vi "(SubVI) Pull DNA_ver2_YCC.vi"(0 "waiting time per point (ms)\nrange from 5ms to 0.167 ms":dbl=0.5, 1 "Filter type":T1(ring), 2 "Avg points":i32, 3 "Real initial position (um)":dbl format="%0.5f", 5 "Record?":bool, 7 "T=X\nF=Y":bool, 9 "Toward  ?\nT=+, F=-":bool, 11 "no Record scan rate  (um/s)":dbl=2.0, 12 "Record scan rate  (um/s)":dbl=2.0 format="%.3f", 13 "range  (um)":dbl=2.0 min=0.0 max=100.0 step=0.5 format="%.3f", 14 "Sampling rate":dbl=20000.0 format="%0.2f") -> (4 "True rate?":bool, 6 "Raw Stage Array":dbl[](array[numeric]), 8 "Filtered Stage Array":dbl[](array[numeric]) format="%0.2f", 10 "Filtered QPD Array":dbl[](array[numeric]) format="%0.2f")   [LabVIEW 2014]
panel:
  out "delay (ms)":dbl
  out "scan rate  (um/s)":dbl
  out "axis":u32=1
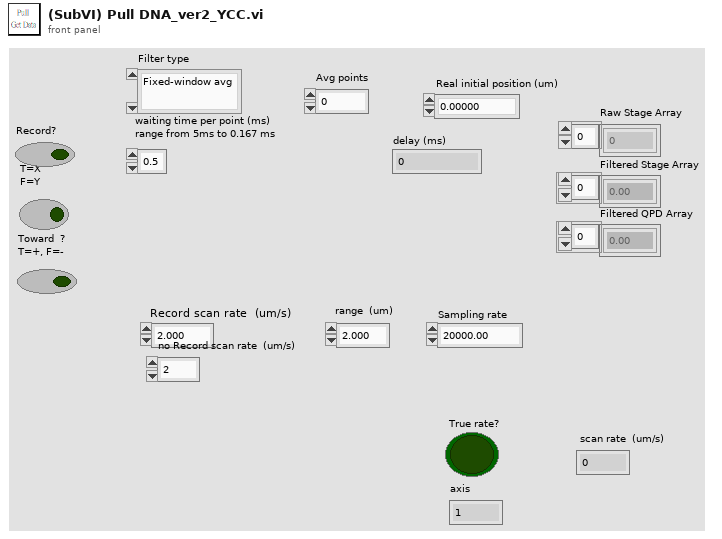
[diagram p1: front panel]
types:
  T1 = enum16{"Fixed-window avg", "Moving-window avg", "F+S-window avg", "S-G filter", "Fixed-window Median", "Moving-window Median "}
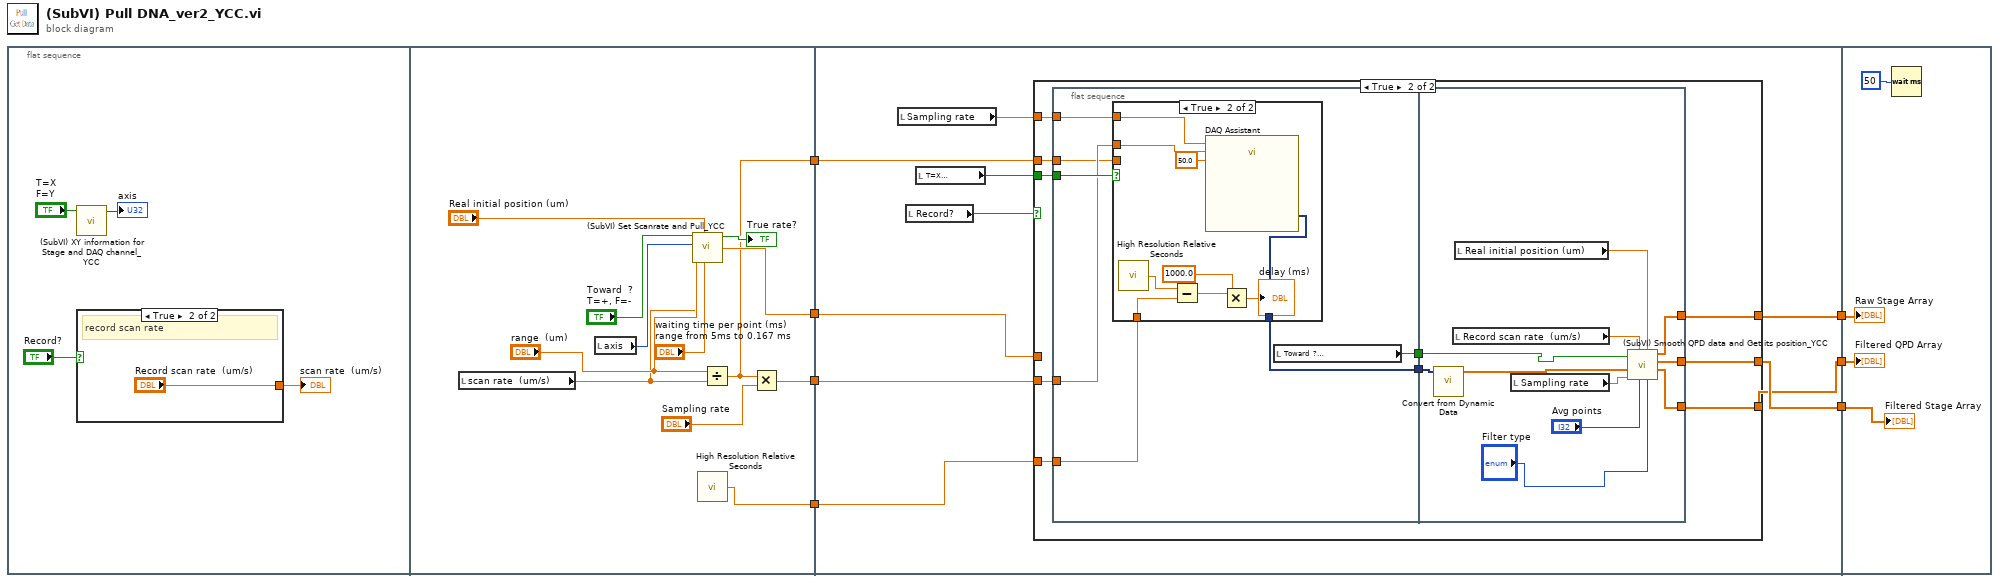
[diagram p0: block diagram]
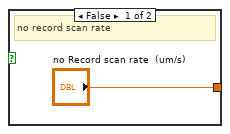
[diagram p2: hidden frame]
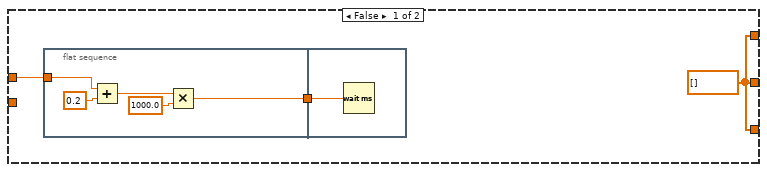
[diagram p3: hidden frame]
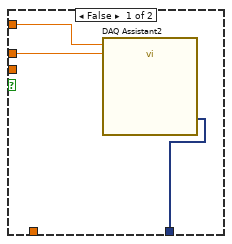
[diagram p4: hidden frame]
diagram:
  n1 = flat-sequence {
    tunnel: [w23] -> w4
    tunnel: [w17] -> w3
    tunnel: [w16] -> w2
    tunnel: [w14] -> w1
    tunnel: [w33] -> w7
    tunnel: [w32] -> w6
    tunnel: [w31] -> w5
    tunnel: w2 -> [w27]
    tunnel: w3 -> [w28]
    tunnel: w4 -> [w35]
    tunnel: w1 -> [w26]
    tunnel: w7 -> [w88]
    tunnel: w6 -> [w87]
    tunnel: w5 -> [w86]
    frame #0 {
      n2 = call "(SubVI) XY information for Stage and DAQ channel_YCC.vi"("T=X\nF=Y"="T=X\nF=Y") -> ("Axis"=→"axis":i32)  [unwired: 3 in, 1 out]
      n3 = case shown="True" "Record?" {
        tunnel: ["no Record scan rate  (um/s)" "Record scan rate  (um/s)"] -> w8
        frame False {
          # "no record scan rate"
        }
        frame True {
          # "record scan rate"
        }
      }
      "scan rate  (um/s)" <- w8
    }
    frame #1 {
      n4 = local read "scan rate  (um/s)"() -> (w18:dbl)
      n5 = local read "axis"() -> (w24:u32)
      n6 = call "(SubVI) Set Scanrate and Pull_YCC.vi"("toward+ ?\nT=+, F=-"="Toward  ?\nT=+, F=-", "Start From  (um)"="Real initial position (um)", "axis"=w24, "scan rate  (um/s)"=w18, "waiting time per point (ms)\nrange from 5ms to 0.167 ms"="waiting time per point (ms)\nrange from 5ms to 0.167 ms", "range  (um)"="range  (um)") -> ("True rate?"=→"True rate?":bool, "traveling time (s)"=w17:dbl)  [unwired: 1 out]
      n7 = call <vilib>:"High Resolution Relative Seconds.vi"() -> ("relative seconds"=w14:dbl)
      n8 = Divide(x="range  (um)", y=w18) -> (x/y=w16:dbl)
      n9 = Multiply(x=w16, y="Sampling rate") -> (x*y=w23:dbl)
    }
    frame #2 {
      n10 = local read "Sampling rate"() -> (w29:dbl)
      n11 = local read "Record?"() -> (w34:bool)
      n12 = local read "T=X\nF=Y"() -> (w30:bool)
      n13 = case shown="True" w34 {
        tunnel: w35 -> [_ w54]
        tunnel: [w38 w51] -> w33
        tunnel: [w38 w50] -> w31
        tunnel: [w38 w49] -> w32
        tunnel: w30 -> [_ w48]
        tunnel: w29 -> [_ w47]
        tunnel: w28 -> [w36 _]
        tunnel: w27 -> [_ w46]
        tunnel: w26 -> [_ w45]
        frame False {
          w38 = dbl[] [] ("data")
          n14 = flat-sequence {
            tunnel: [w42] -> w37
            tunnel: w36 -> [w39]
            tunnel: w37 -> [w44]
            frame #0 {
              n15 = Add(x=w39, y=0.2) -> (x+y=w40:dbl)
              n16 = Multiply(x=w40, y=1000.0) -> (x*y=w42:dbl)
            }
            frame #1 {
              n17 = Wait (ms)(milliseconds to wait=w44) -> ()  [unwired: 1 out]
            }
          }
        }
        frame True {
          n18 = flat-sequence {
            tunnel: w54 -> [w57]
            tunnel: [w61] -> w53
            tunnel: [w58] -> w52
            tunnel: w48 -> [w60]
            tunnel: w47 -> [w59]
            tunnel: w46 -> [w56]
            tunnel: w45 -> [w55]
            tunnel: w53 -> [w76]
            tunnel: w52 -> [w80]
            tunnel: [w79] -> w51
            tunnel: [w78] -> w50
            tunnel: [w77] -> w49
            frame #0 {
              n19 = case shown="True" w60 {
                tunnel: w59 -> [w64 w73]
                tunnel: [w63 w71] -> w58
                tunnel: w57 -> [w62 w72]
                tunnel: w56 -> [_ _]
                tunnel: w55 -> [_ w66]
                frame False {
                  n20 = call "DAQ Assistant2"("rate"=w64, "number of samples"=w62) -> ("data"=w63:dynamicdata)  [unwired: 15 in, 2 out]
                }
                frame True {
                  n21 = call <vilib>:"High Resolution Relative Seconds.vi"() -> ("relative seconds"=w70:dbl)
                  n22 = Subtract(x=w70, y=w66) -> (x-y=w69:dbl)
                  n23 = call "DAQ Assistant"("rate"=w73, "number of samples"=w72, "timeout (s)"=50.0) -> ("data"=w71:dynamicdata)  [unwired: 14 in, 2 out]
                  n24 = Multiply(x=w69, y=1000.0) -> (x*y=→"delay (ms)":dbl)
                }
              }
              n25 = local read "Toward  ?\nT=+, F=-"() -> (w61:bool)
            }
            frame #1 {
              n26 = call "Convert from Dynamic Data"("Dynamic Data Type"=w80) -> ("Array"=w75:dbl[])  [unwired: 3 in]
              n27 = local read "Record scan rate  (um/s)"() -> (w81:dbl)
              n28 = local read "Real initial position (um)"() -> (w84:dbl)
              n29 = local read "Sampling rate"() -> (w83:dbl)
              n30 = call "(SubVI) Smooth QPD data and Get its position_YCC.vi"("Filter type"="Filter type", "Initial position (um)"=w84, "Avg points"="Avg points", "scan rate  (um/s)"=w81, "Sampling rate (Hz)"=w83, "QPD data"=w75, "Direction\nT=+ \nF=-"=w76) -> ("Filtered QPD data"=w78:dbl[], "Filtered Stage Array"=w77:dbl[], "Raw Stage Array"=w79:dbl[])  [unwired: 2 in]
            }
          }
        }
      }
    }
    frame #3 {
      n31 = Wait (ms)(milliseconds to wait=u32 50) -> ()  [unwired: 1 out]
      "Raw Stage Array" <- w88
      "Filtered Stage Array" <- w87
      "Filtered QPD Array" <- w86
    }
  }
